vi "UHR-Fleezers Control (host) - 12.1.vi"() -> ()   [LabVIEW 2012] (continued)
            n683 = property on="Trap Pos. FB Offset Factor" class="DigNum (strict)"("Val(Sgnl)"=i64 0 ("Value (Signaling)")) -> ()  [unwired: 2 in, 2 out]
            n684 = local write "Stage Moving"(TRUE ("Stage Moving")) -> ()
            n685 = call "move to saved stage position.vi"("error in"=w1101, "Stage VISA resource name in"=w1102, "Position"="Stage Position To Establish FB", "Saved Stage Positions"=w1104) -> ("error out"=w1100:errorcluster)  [unwired: 1 out]
            n686 = local write "Stage Control Serial Error"(w1100) -> ()
          }
          frame #2 {
            n687 = call <vilib>:"Beep.vi"() -> ()  [unwired: 3 in, 9 out]
            n688 = Multiply(x="Wait (s)", y=u32 1000 ("milliseconds to wait")) -> (x*y=w1111:u32)
            n689 = property on="Trap Delta (MHz)" class="DigNum (strict)"("Val(Sgnl)"="Starting \nTrap Delta (MHz)") -> ()  [unwired: 2 in, 2 out]
            n690 = local write "Stage Moving"(FALSE ("Stage Moving")) -> ()
            n691 = Wait (ms)(milliseconds to wait=w1111) -> ()  [unwired: 1 out]
            n692 = property on="Tab Control 2" class="TabCtl (strict)"("Val(Sgnl)"=T6."Feedback on Trap Position" ("Value (Signaling)")) -> ()  [unwired: 2 in, 2 out]
            n693 = property on="Tab Control" class="TabCtl (strict)"("Val(Sgnl)"=T4."Trap Control (RF)" ("Value (Signaling)")) -> ()  [unwired: 2 in, 2 out]
          }
          frame #3 {
            n694 = property on="Set Reading to\nSetpoint" class="Bool (strict)"("Val(Sgnl)"=TRUE ("Value (Signaling)")) -> ()  [unwired: 2 in, 2 out]
            n695 = Wait (ms)(milliseconds to wait=u32 500) -> ()  [unwired: 1 out]
          }
          frame #4 {
            n696 = property on="Trap Pos. FB ON" class="Bool (strict)"("Val(Sgnl)"=TRUE ("Value (Signaling)")) -> ()  [unwired: 2 in, 2 out]
            n697 = Wait (ms)(milliseconds to wait=u32 250) -> ()  [unwired: 1 out]
          }
          frame #5 {
            n698 = case shown="False" "Trap Trig Fl." {
              frame False {
                n699 = case shown="True" "Green ON after FB ON?" {
                  selector: "Green ON after FB ON?" -> [_ w1126]
                  frame False {
                  }
                  frame True {
                    n700 = property on="Green Laser ON/Interlacing" class="Bool (strict)"("Val(Sgnl)"=w1126) -> ()  [unwired: 2 in, 2 out]
                  }
                }
              }
              frame True {
              }
            }
            n701 = case shown="True" "Remove Action Offset" {
              tunnel: TRUE ("Value (Signaling)") -> [w1123 w1124]
              frame False {
                n702 = property on="Remove Unwinding Offset" class="Bool (strict)"("Val(Sgnl)"=w1123) -> ()  [unwired: 2 in, 2 out]
              }
              frame True {
                n703 = property on="Remove Action Offset" class="Bool (strict)"("Val(Sgnl)"=w1124) -> ()  [unwired: 2 in, 2 out]
              }
            }
            n704 = Wait (ms)(milliseconds to wait=u32 250) -> ()  [unwired: 1 out]
          }
          frame #6 {
            n705 = property on="Start Saving" class="Bool (strict)"("Val(Sgnl)"=TRUE ("Value (Signaling)")) -> ()  [unwired: 2 in, 2 out]
            n706 = Wait (ms)(milliseconds to wait=u32 5000) -> ()  [unwired: 1 out]
          }
          frame #7 {
            w1130 = TRUE ("Value (Signaling)")
            n707 = property on="Rem fb disp offset" class="Bool (strict)"("Val(Sgnl)"=w1130) -> ()  [unwired: 2 in, 2 out]
            n708 = property on="Remove Offset" class="Bool (strict)"("Val(Sgnl)"=w1130) -> ()  [unwired: 2 in, 2 out]
            n709 = Wait (ms)(milliseconds to wait=u32 100) -> ()  [unwired: 1 out]
          }
          frame #8 {
            n710 = case shown="True" w1133 {
              frame False {
              }
              frame True {
                n711 = local write "Trap Trig. Fl."(TRUE ("Value (Signaling)")) -> ()
              }
            }
          }
          frame #9 {
            n712 = case shown="True" "Start dipping after?" {
              frame False {
              }
              frame True {
                n713 = flat-sequence {
                  frame #0 {
                    n714 = Multiply(x="Delay before dipping (s)", y=1000.0) -> (x*y=w1137:dbl)
                    n715 = Wait (ms)(milliseconds to wait=w1137) -> ()  [unwired: 1 out]
                  }
                  frame #1 {
                    n716 = property on="Dip for Protein" class="Bool (strict)"("Val(Sgnl)"=TRUE ("Value (Signaling)")) -> ()  [unwired: 2 in, 2 out]
                    n717 = local write "Scripts"(T1."Dipping" ("Scripts")) -> ()
                  }
                }
              }
            }
          }
        }
      }
      event "Fixed Traps Data\nScript": Value Change {
        n718 = event-data() -> ()  [unwired: 1 in, 5 out]
        n719 = flat-sequence {
          frame #0 {
            n720 = case shown="True" "Green ON" {
              frame False {
              }
              frame True {
                n721 = property on="Green Laser ON/Interlacing" class="Bool (strict)"("Val(Sgnl)"=TRUE) -> ()  [unwired: 2 in, 2 out]
              }
            }
            n722 = local write "Offset (nm)"(0.0 ("Offset (nm)")) -> ()
            n723 = property on="Sample Channel\nFlow" class="Bool (strict)"("Val(Sgnl)"=FALSE ("Value (Signaling)")) -> ()  [unwired: 2 in, 2 out]
            n724 = property on="Trap Delta (MHz)" class="DigNum (strict)"("Val(Sgnl)"="Fixed Traps Trap Delta (MHz)") -> ()  [unwired: 2 in, 2 out]
          }
          frame #1 {
            n725 = Wait (ms)(milliseconds to wait=u32 1000) -> ()  [unwired: 1 out]
          }
          frame #2 {
            n726 = local write "Start Saving"(TRUE ("Start Saving")) -> ()
          }
          frame #3 {
            n727 = local read "Bead Sep. Int. Time (s)"() -> (w1148:dbl)
            n728 = Multiply(x=w1148, y=1000.0) -> (x*y=w1150:dbl)
            n729 = Wait (ms)(milliseconds to wait=w1150) -> ()  [unwired: 1 out]
          }
          frame #4 {
            n730 = property on="Remove Offset" class="Bool (strict)"("Val(Sgnl)"=TRUE ("Value (Signaling)")) -> ()  [unwired: 2 in, 2 out]
          }
          frame #5 {
            n731 = property on="Dip for Protein" class="Bool (strict)"("Val(Sgnl)"="Start dipping after?") -> ()  [unwired: 2 in, 2 out]
          }
        }
      }
      event "Got DNA bead": Value Change {
        n732 = event-data() -> ()  [unwired: 1 in, 5 out]
        n733 = flat-sequence {
          frame #0 {
            n734 = local read "Daq spot flow on"() -> (w1155:bool)
            n735 = case shown="True" w1155 {
              frame False {
              }
              frame True {
                n736 = property on="Sample Channel\nFlow" class="Bool (strict)"("Val(Sgnl)"=TRUE ("Value (Signaling)")) -> ()  [unwired: 2 in, 2 out]
              }
            }
            n737 = property on="Got DNA bead" class="Bool"("Key Focus"=FALSE) -> ()  [unwired: 2 in, 2 out]
          }
          frame #1 {
            n738 = property on="Inject Pump 1" class="Bool (strict)"("Val(Sgnl)"=FALSE ("Value (Signaling)")) -> ()  [unwired: 2 in, 2 out]
          }
          frame #2 {
            n739 = property on="Cal/Data Acq. Spot" class="Bool (strict)"("Val(Sgnl)"=TRUE ("Value (Signaling)")) -> ()  [unwired: 2 in, 2 out]
          }
        }
      }
      event "Take Stepping Data": Value Change {
        n740 = event-data() -> ()  [unwired: 1 in, 5 out]
        n741 = local read "Save ave N"() -> (w1167:dbl)
        n742 = flat-sequence {
          tunnel: w1167 -> [w1169]
          tunnel: [w1169] -> w1162
          tunnel: [w1171] -> w1163
          tunnel: w1162 -> [w1171]
          tunnel: [w1173] -> w1164
          tunnel: w1163 -> [w1173]
          tunnel: [w1176] -> w1165
          tunnel: w1164 -> [w1176]
          tunnel: [w1178] -> w1166
          tunnel: w1165 -> [w1178]
          tunnel: [w1180] -> w1160
          tunnel: w1166 -> [w1180]
          tunnel: w1160 -> [w1183]
          tunnel: [w1183] -> w1159
          tunnel: w1159 -> [w1184]
          tunnel: [w1184] -> w1161
          tunnel: w1161 -> [w1190]
          frame #0 {
            n743 = property on="Save ave N" class="DigNum (strict)"("Val(Sgnl)"="Save ave factor") -> ()  [unwired: 2 in, 2 out]
          }
          frame #1 {
            n744 = Wait (ms)(milliseconds to wait=u32 100) -> ()  [unwired: 1 out]
          }
          frame #2 {
            n745 = local read "Offset 2 Start (MHz)"() -> (w1175:dbl)
            n746 = property on="Saved AOD Raster Scan Parameter Sets" class="Arr (strict)"("Index Values"=u32[] [2]) -> ()  [unwired: 2 in, 2 out]
            n747 = property on="Trap Delta (MHz)" class="DigNum (strict)"("Val(Sgnl)"=w1175) -> ()  [unwired: 2 in, 2 out]
          }
          frame #3 {
            n748 = property on="Load parameters" class="Bool (strict)"("Val(Sgnl)"=TRUE ("Value (Signaling)")) -> ()  [unwired: 2 in, 2 out]
          }
          frame #4 {
            n749 = Wait (ms)(milliseconds to wait=u32 100) -> ()  [unwired: 1 out]
          }
          frame #5 {
            n750 = property on="Trap Raster Scan" class="Bool (strict)"("Val(Sgnl)"=TRUE ("Value (Signaling)")) -> ()  [unwired: 2 in, 2 out]
          }
          frame #6 {
            n751 = Wait (ms)(milliseconds to wait=u32 1000) -> ()  [unwired: 1 out]
          }
          frame #7 {
            n752 = while {
              stop <- w1187 stop-if-true
              n753 = local read "Raster Scanning..."() -> (w1189:bool)
              n754 = local read "Saving..."() -> (w1188:bool)
              n755 = Not(x=w1188) -> (.not. x?=w1185:bool)
              n756 = Not(x=w1189) -> (.not. x?=w1186:bool)
              n757 = And(x=w1186, y=w1185) -> (x .and. y?=w1187:bool)
            }
          }
          frame #8 {
            n758 = property on="Save ave N" class="DigNum (strict)"("Val(Sgnl)"=w1190) -> ()  [unwired: 2 in, 2 out]
          }
        }
      }
      event "Step Size (nm)": Value Change {
        n759 = event-data() -> ()  [unwired: 1 in, 5 out]
        n760 = flat-sequence {
          frame #0 {
            n761 = property on="Saved AOD Raster Scan Parameter Sets" class="Arr (strict)"("Index Values"=u32[] [1]) -> ()  [unwired: 2 in, 2 out]
          }
          frame #1 {
            n762 = Multiply(x="N Steps", y="Step Size (nm)") -> (x*y=w1192:dbl)
            n763 = property on="Scan Speed AOD (nm/s) 2" class="DigNum (strict)"("Value"="Step Size (nm)") -> ()  [unwired: 2 in, 2 out]
            n764 = property on="Step Size AOD (nm) 2" class="DigNum (strict)"("Value"="Step Size (nm)") -> ()  [unwired: 2 in, 2 out]
            n765 = property on="Scan Range AOD (nm) 2" class="DigNum (strict)"("Value"=w1192) -> ()  [unwired: 2 in, 2 out]
          }
        }
      }
      event "Take Detection Laser\nImage": Value Change {
        n766 = event-data() -> ()  [unwired: 1 in, 5 out]
        n767 = flat-sequence {
          tunnel: [w1220] -> w1210
          tunnel: [w1219] -> w1203
          tunnel: [w1218] -> w1195
          tunnel: [w1223] -> w1211
          tunnel: w1210 -> [w1223]
          tunnel: [w1222] -> w1204
          tunnel: w1203 -> [w1222]
          tunnel: [w1221] -> w1196
          tunnel: w1195 -> [w1221]
          tunnel: [w1227] -> w1212
          tunnel: w1211 -> [w1227]
          tunnel: [w1226] -> w1205
          tunnel: w1204 -> [w1226]
          tunnel: [w1225] -> w1197
          tunnel: w1196 -> [w1225]
          tunnel: [w1233] -> w1213
          tunnel: w1212 -> [w1233]
          tunnel: [w1232] -> w1206
          tunnel: w1205 -> [w1232]
          tunnel: [w1231] -> w1198
          tunnel: w1197 -> [w1231]
          tunnel: [w1237] -> w1214
          tunnel: w1213 -> [w1237]
          tunnel: [w1236] -> w1207
          tunnel: w1206 -> [w1236]
          tunnel: [w1235] -> w1199
          tunnel: w1198 -> [w1235]
          tunnel: [w1241] -> w1215
          tunnel: w1214 -> [w1241]
          tunnel: [w1240] -> w1208
          tunnel: w1207 -> [w1240]
          tunnel: [w1239] -> w1200
          tunnel: w1199 -> [w1239]
          tunnel: [w1245] -> w1216
          tunnel: w1215 -> [w1245]
          tunnel: [w1244] -> w1209
          tunnel: w1208 -> [w1244]
          tunnel: [w1243] -> w1201
          tunnel: w1200 -> [w1243]
          tunnel: w1216 -> [w1251]
          tunnel: w1209 -> [w1250]
          tunnel: [w1248] -> w1202
          tunnel: w1201 -> [w1248]
          tunnel: w1202 -> [w1252]
          frame #0 {
            n768 = local read "Green Laser ON/Interlacing"() -> (w1220:bool)
            n769 = local read "Green laser mode"() -> (w1219:enum32{"Laser ON", "Laser OFF", "Interlace"})
            n770 = local read "Green FB On/Off"() -> (w1218:bool)
          }
          frame #1 {
            n771 = property on="Green FB On/Off" class="Bool (strict)"("Val(Sgnl)"=FALSE ("Value (Signaling)")) -> ()  [unwired: 2 in, 2 out]
          }
          frame #2 {
            n772 = property on="Green Laser ON/Interlacing" class="Bool (strict)"("Val(Sgnl)"=TRUE ("Value (Signaling)")) -> ()  [unwired: 2 in, 2 out]
            n773 = property on="Flip Green Filter" class="Bool (strict)"("Val(Sgnl)"=TRUE ("Value (Signaling)")) -> ()  [unwired: 2 in, 2 out]
            n774 = property on="Green laser mode" class="RadioBtnsControl (strict)"("Val(Sgnl)"=enum32{"Laser ON", "Laser OFF", "Interlace"}."Laser ON" ("Value (Signaling)")) -> ()  [unwired: 2 in, 2 out]
          }
          frame #3 {
            n775 = Wait (ms)(milliseconds to wait=u32 500) -> ()  [unwired: 1 out]
          }
          frame #4 {
            n776 = property on="Confocal Image" class="Bool (strict)"("Val(Sgnl)"=TRUE ("Value (Signaling)")) -> ()  [unwired: 2 in, 2 out]
          }
          frame #5 {
            n777 = Wait (ms)(milliseconds to wait=u32 2000) -> ()  [unwired: 1 out]
          }
          frame #6 {
            n778 = while {
              stop <- w1246 stop-if-true
              n779 = local read "Saving..."() -> (w1247:bool)
              n780 = Not(x=w1247) -> (.not. x?=w1246:bool)
            }
          }
          frame #7 {
            n781 = property on="Flip Green Filter" class="Bool (strict)"("Val(Sgnl)"=TRUE ("Value (Signaling)")) -> ()  [unwired: 2 in, 2 out]
            n782 = property on="Green Laser ON/Interlacing" class="Bool (strict)"("Val(Sgnl)"=w1251) -> ()  [unwired: 2 in, 2 out]
            n783 = property on="Green laser mode" class="RadioBtnsControl (strict)"("Val(Sgnl)"=w1250) -> ()  [unwired: 2 in, 2 out]
          }
          frame #8 {
            n784 = property on="Green FB On/Off" class="Bool (strict)"("Val(Sgnl)"=w1252) -> ()  [unwired: 2 in, 2 out]
          }
        }
      }
      event "Stop All": Value Change {
        n785 = event-data() -> ()  [unwired: 1 in, 5 out]
        n786 = local read "Stop All"() -> (w1253:bool)
      }
    }
    n787 = node-c288() -> ()  [unwired: 1 in, 1 out]
  }
  n788 = node-c288(3 ("Processor")) -> (w114:T20)  [unwired: 3 out]
  n789 = flat-sequence "Video" {
    tunnel: [w1263] -> w104
    tunnel: w104 -> [w1303]
    frame #0 {
      n790 = while {
        stop <- w1255 continue-if-true
        n791 = call "Close Video Capture.vi"() -> ("error code OUT"=w1257:i32)
        n792 = Equal?(x=w1257, y=0) -> (x = y?=w1255:bool)
      }
      n793 = local write "Stop All"(FALSE ("Stop All")) -> ()
    }
    frame #1 {
      n794 = call "DMR_Init.vi"() -> ()  [unwired: 3 out]
    }
    frame #2 {
      w1258 = "DE245428202"  # MSU fleezers card #
      (unwired) "DE019116701"  # Illinois fleezers card #
      # "Setting the destination format to Mono8 makes sure that the image can be displayed in the intensity plot."
      n795 = call "DMR_GetDevice.vi"("search string IN"=w1258) -> ("device handle OUT"=w1281:i32)  [unwired: 4 in, 2 out]
      n796 = call "DMR_OpenDevice.vi"("device handle IN"=w1281) -> ("driver handle OUT"=w1264:i32)  [unwired: 4 out]
      n797 = call "DMR_FindList.vi"("flags IN"=u32 0 ("flags"), "list name IN"="" ("String"), "list type IN"=T25."camera descriptions", "driver handle IN"=w1264) -> ("list handle OUT"=w1267:i32)  [unwired: 2 out]
      n798 = call "DMR_FindList.vi"("flags IN"=u32 0 ("flags"), "list name IN"="Base", "list type IN"=T25."setting", "driver handle IN"=w1264) -> ("list handle OUT"=w1265:i32)  [unwired: 2 out]
      n799 = call "OBJ_GetHandle.vi"("object name IN"="VideoStandard", "list handle IN"=w1267) -> ("object handle OUT"=w1261:i32)  [unwired: 3 out]
      n800 = call "OBJ_GetHandle.vi"("object name IN"="PixelFormat", "list handle IN"=w1265) -> ("object handle OUT"=w1275:i32)  [unwired: 3 out]
      n801 = call "OBJ_SetS.vi"("value index IN"=0, "value IN"="NTSC M", "object handle IN"=w1261) -> ()  [unwired: 2 out]
      n802 = call "OBJ_SetS.vi"("value index IN"=0, "value IN"="Mono8" ("value"), "object handle IN"=w1275) -> ()  [unwired: 2 out]
      n803 = call "OBJ_GetHandle.vi"("object name IN"="VideoChannel", "list handle IN"=w1265) -> ("object handle OUT"=w1271:i32)  [unwired: 3 out]
      n804 = while {
        tunnel: [w1285] -> w1263
        tunnel: w1264 -> [w1282]
        stop <- w1283 continue-if-true
        n805 = call "DMR_ImageRequestSingle.vi"("request control IN"=0, "driver handle IN"=w1282) -> ("error code OUT"=w1284:i32, "driver handle OUT"=w1285:i32)  [unwired: 2 out]
        n806 = Equal To 0?(x=w1284) -> (x = 0?=w1283:bool)
      }
      n807 = call "OBJ_SetI.vi"("value index IN"=0, "value IN"=3 ("Video channel"), "object handle IN"=w1271) -> ()  [unwired: 2 out]
    }
    frame #3 {
      w1291 = T16 0 items=["Grayscale (U8)", "Grayscale (I16)", "Grayscale (SGL)", "Complex (CSG)", "RGB (U32)", "HSL (U32)", "RGB (U64)"] ("Image Type")
      w1299 = T16 0 items=["Grayscale (U8)", "Grayscale (I16)", "Grayscale (SGL)", "Complex (CSG)", "RGB (U32)", "HSL (U32)", "RGB (U64)"] ("Image Type")
      n808 = for "Create Greyscale map" {
        N: 256 -> [_]
        tunnel: [w1305] -> w1288 mode=indexing
        workers-P: _ -> [_]
        i -> [w1308]
        n809 = To Unsigned Byte Integer(number=w1308) -> (unsigned 8bit integer=w1304:u8)
        n810 = Join Numbers(hi=w1304, lo=w1304) -> ((hi.lo)=w1307:u16)
        n811 = Join Numbers(hi=w1304, lo=w1304) -> ((hi.lo)=w1306:u16)
        n812 = Join Numbers(hi=w1307, lo=w1306) -> ((hi.lo)=w1305:u32)
      }
      n813 = call "IMAQ Create"("Image Name"="Scaled video", "Image Type"=w1291) -> ("New Image"=w1290:T2)  [unwired: 2 in, 2 out]
      n814 = call "IMAQ Create"("Image Name"="Main video", "Image Type"=w1299) -> ("New Image"=w1300:T2)  [unwired: 2 in, 2 out]
      n815 = node-c288(0 ("Processor")) -> (w1298:T20)  [unwired: 3 out]
      n816 = Initialize Array(u32 0 ("Window Number (0...15)"), 480 ("dimension size"), 640 ("dimension size")) -> (w1293:u32[][])
      n817 = timed-loop {
        tunnel: w1303 -> [w1325]
        tunnel: [w1324] -> w1302
        tunnel: w1300 -> [w1323]
        timing: w1298 -> [_]
        timing-out: [_] -> w1297
        tunnel: w1293 -> [w1312]
        tunnel: w1290 -> [w1310]
        tunnel: w1288 -> [w1309]
        stop <- w1311 stop-if-true
        # "This block performs the \nactual image capture."
        n818 = node-c288() -> ()  [unwired: 2 out]
        n819 = local read "Stop All"() -> (w1311:bool)
        n820 = Reciprocal(x="Video Capture Rate (Hz)") -> (1/x=w1315:dbl)
        n821 = Multiply(x=w1315, y=1000.0) -> (x*y=w1313:dbl)
        n822 = call "DMR_ImageRequestWaitFor.vi"("queue number IN"=0, "timeout(ms) IN"=500, "driver handle IN"=w1325) -> ("error code OUT"=w1329:i32, "request number OUT"=w1326:i32, "driver handle OUT"=w1327:i32)
        n823 = feedback #1(T26 refnum ("Avi Refnum")) -> (w1317:T26)
        n824 = case shown="True" "New Video File" {
          tunnel: [T26 refnum ("Avi Refnum") w1346] -> w1319
          tunnel: [FALSE TRUE] -> w1320
          tunnel: w1317 -> [_ w1342]
          frame False {
          }
          frame True {
            n825 = call "Create new save file.vi"("Ext"=".avi" ("string"), "Index In"="Video Index") -> ("Path Out"=w1338:path, "Index Out"=w1339:dbl)  [unwired: 1 in]
            "Path Out" <- w1338
            n826 = Not Equal?(x=w1342, y=T26 refnum ("Avi Refnum")) -> (x != y?=w1343:bool)
            n827 = Increment(x=w1339) -> (x+1=w1348:dbl)
            n828 = case shown="True" w1343 {
              tunnel: w1342 -> [_ w1349]
              frame False {
              }
              frame True {
                n829 = call "IMAQ AVI Close"("Avi Refnum"=w1349) -> ()  [unwired: 1 in, 10 out]
              }
            }
            n830 = local write "Video Index"(w1348) -> ()
            n831 = call "IMAQ AVI Create"("Frames Per Second"=u32 30, "AVI Path"=w1338) -> ("Avi Refnum"=w1346:T26)  [unwired: 5 in, 4 out]
          }
        }
        n832 = Equal To 0?(x=w1329) -> (x = 0?=w1328:bool)
        n833 = Select(t=w1319, s=w1320, f=w1317) -> (s? t:f=w1318:T26)
        n834 = feedback-in #1(w1318) -> ()
        n835 = case shown="True" w1328 {
          tunnel: w1327 -> [w1350 w1375]
          tunnel: w1326 -> [_ w1374]
          tunnel: [w1350 w1371] -> w1324
          tunnel: w1323 -> [_ w1355]
          tunnel: w1312 -> [_ w1359]
          tunnel: w1318 -> [_ w1357]
          tunnel: w1310 -> [_ w1352]
          tunnel: w1309 -> [_ w1351]
          frame False {
          }
          frame True {
            w1365 = u32 0 ("X-offset IN")
            n836 = call "DMR_GetImageRequestBufferData.vi"("driver handle IN"=w1375, "request number IN"=w1374) -> ("width OUT"=w1364:i32, "height OUT"=w1363:i32, "driver handle OUT"=w1370:i32, "request number OUT"=w1369:i32, "bytes per pixel OUT"=w1366:i32)  [unwired: 13 out]
            n837 = call "DMR_GetImageRequestBufferImageData.vi"("driver handle IN"=w1370, "request number IN"=w1369, "bytes per pixel IN"=w1366, "X-offset IN"=w1365, "Y-offset IN"=w1365, "height IN"=w1363, "width IN"=w1364) -> ("driver handle OUT"=w1368:u32, "request number OUT"=w1367:u32, "image OUT"=w1360:u32[][])  [unwired: 10 out]
            n838 = call "DMR_ImageRequestUnlock.vi"("request number IN"=w1367, "driver handle IN"=w1368) -> ("driver handle OUT"=w1373:i32)  [unwired: 1 in, 2 out]
            n839 = case shown="True" "Averaging" {
              tunnel: w1360 -> [w1411 w1416]
              tunnel: [w1411 w1415] -> w1356
              tunnel: w1359 -> [_ w1413]
              frame False {
              }
              frame True {
                (unwired) 1
                w1421 = 1
                n840 = feedback #2(w1413) -> (w1412:u32[][])
                n841 = Add(x=w1416, y=w1412) -> (x+y=w1417:u32[][])
                n842 = Select(t=w1413, s="Reset Averaging", f=w1417) -> (s? t:f=w1419:u32[][])
                n843 = feedback-in #2(w1419) -> ()
                n844 = feedback #3(w1421) -> (w1414:i32)
                n845 = Divide(x=w1417, y=w1414) -> (x/y=w1418:dbl[][])
                n846 = Increment(x=w1414) -> (x+1=w1422:i32)
                n847 = To Unsigned Long Integer(number=w1418) -> (unsigned 32bit integer=w1415:u32[][])
                n848 = Select(t=w1421, s="Reset Averaging", f=w1422) -> (s? t:f=w1420:i32)
                n849 = feedback-in #3(w1420) -> ()
              }
            }
            n850 = call "DMR_ImageRequestSingle.vi"("request control IN"=0, "driver handle IN"=w1373) -> ("driver handle OUT"=w1371:i32)  [unwired: 3 out]
            n851 = disable-structure shown="Disabled" {
              disable-tunnel: w1356 -> [w1388 _]
              disable-tunnel: w1352 -> [w1387 _]
              frame Disabled {
                n852 = To Double Precision Float(number=w1388) -> (double precision float=w1386:dbl[][])
                n853 = In Range and Coerce(upper limit="Intensity Upper", x=w1386, lower limit="Intensity Lower") -> (coerced(x)=w1385:dbl[][])  [unwired: 1 out]
                n854 = Subtract(x="Intensity Upper", y="Intensity Lower") -> (x-y=w1382:dbl)
                n855 = Subtract(x=w1385, y="Intensity Lower") -> (x-y=w1383:dbl[][])
                n856 = Divide(x=w1383, y=w1382) -> (x/y=w1384:dbl[][])
                n857 = Multiply(x=255.0, y=w1384) -> (x*y=w1380:dbl[][])
                n858 = To Unsigned Byte Integer(number=w1380) -> (unsigned 8bit integer=w1389:u8[][])
                n859 = call "IMAQ ArrayToImage"("Image Pixels (U8)"=w1389, "Image"=w1387) -> ("Image Out"=w1376:T2)  [unwired: 4 in, 5 out]
                n860 = First Call?() -> (First Call?: T/F=w1377:bool)
                n861 = case shown="True" w1377 {
                  tunnel: w1376 -> [w1390 w1401]
                  frame False {
                    n862 = flat-sequence {
                      tunnel: w1390 -> [w1396]
                      frame #0 {
                        w1393 = FALSE ("Get/Set Status? (Set)")
                        w1392 = 0 ("Window Number (0...15)")
                        n863 = call "IMAQ WindSize"("Get/Set Status? (Set)"=w1393, "Window Number"=w1392) -> ("Width & Height out"=→"Window Size":cluster{"Width":i32, "Height":i32})  [unwired: 4 in, 2 out]
                        n864 = call "IMAQ WindMove"("Window Number (0...15)"=w1392, "Get/Set Status? (Set)"=w1393) -> ("Coordinates (screen)"=→"Window Position":cluster{"X Position":i32, "Y Position":i32})  [unwired: 3 in, 1 out]
                        n865 = call "IMAQ WindDraw"("Resize to Image Size? (Y)"=FALSE, "Window Number (0...15)"=w1392, "Image"=w1396) -> ()  [unwired: 7 in, 2 out]
                      }
                      frame #1 {
                        n866 = call "IMAQ WindZoom 2"("Center Point"="Center Point", "Zoom to Fit? (False)"=FALSE, "Zoom Factor"="Zoom Factor") -> ()  [unwired: 5 in, 4 out]
                      }
                    }
                  }
                  frame True {
                    n867 = flat-sequence {
                      tunnel: w1401 -> [w1404]
                      tunnel: [w1402] -> w1400
                      tunnel: w1400 -> [w1406]
                      frame #0 {
                        w1403 = TRUE ("Resize to Image Size? (Y)")
                        w1402 = 0 ("Window Number (0...15)")
                        n868 = call "IMAQ WindNonTearing"("Window Number"=w1402, "NonTearing? (True)"=w1403) -> ()  [unwired: 8 in, 2 out]
                        n869 = call "IMAQ WindDraw"("Resize to Image Size? (Y)"=w1403, "Window Number (0...15)"=w1402, "Image"=w1404) -> ()  [unwired: 7 in, 2 out]
                      }
                      frame #1 {
                        n870 = call "IMAQ WindSize"("Scrollbars? (N)"=FALSE, "Width & Height"="Initial Window Size", "Window Number"=w1406) -> ()  [unwired: 3 in, 3 out]
                        n871 = call "IMAQ WindMove"("Window Number (0...15)"=w1406, "Coordinates (screen)"="Initial Window Position") -> ()  [unwired: 3 in, 2 out]
                      }
                    }
                  }
                }
              }
              frame Enabled {
              }
            }
            n872 = To Unsigned Byte Integer(number=w1356) -> (unsigned 8bit integer=w1354:u8[][])
            n873 = call "IMAQ ArrayToImage"("Image Pixels (U8)"=w1354, "Image"=w1355) -> ("Image Out"=w1353:T2)  [unwired: 4 in, 5 out]
            "Primary Video Display" <- w1353
            n874 = case shown="True" "Save Video" {
              tunnel: w1357 -> [_ w1410]
              tunnel: w1353 -> [_ w1409]
              frame False {
              }
              frame True {
                n875 = call "IMAQ AVI Write Frame"("Image"=w1409, "Avi Refnum"=w1410) -> ()  [unwired: 2 in, 8 out]
              }
            }
            n876 = case shown="True" "Save Image" {
              tunnel: w1354 -> [_ w1425]
              tunnel: w1351 -> [_ w1424]
              frame False {
              }
              frame True {
                n877 = call <vilib>:"Flatten Pixmap.vi"("colors"=w1424, "8-bit pixmap"=w1425) -> ("image data"=w1431:T27)  [unwired: 4 in, 5 out]
                n878 = call "Create new save file.vi"("Insert"="video_frame_" ("string"), "Ext"=".bmp" ("string"), "Index In"="Image Index") -> ("Path Out"=w1427:path, "Index Out"=w1432:dbl)
                n879 = Increment(x=w1432) -> (x+1=w1426:dbl)
                n880 = local write "Image Index"(w1426) -> ()
                n881 = call <vilib>:"Write BMP File.vi"("image data"=w1431, "path to BMP file"=w1427) -> ()  [unwired: 1 in, 9 out]
              }
            }
          }
        }
        n882 = node-c288(w1313) -> ()  [unwired: 1 out]
      }
      n883 = node-c288(w1297) -> ()  [unwired: 1 out]
      n884 = call "DMR_CloseDevice.vi"("driver handle IN"=w1302) -> ()  [unwired: 1 in, 4 out]
    }
    frame #4 {
      n885 = call "DMR_Close.vi"() -> ()  [unwired: 1 out]
    }
  }
  n886 = timed-loop "Acquire Data" {
    tunnel: w28 -> [w1724]
    tunnel: w76 -> [w1723]
    tunnel: [w1753] -> w286
    tunnel: [w1748] -> w284
    timing: w194 -> [_]
    timing-out: [_] -> w193
    tunnel: w93 -> [w1569]
    stop <- "Stop All" stop-if-true
    w1484 = "Initialize"
    w1554 = "NI_ChannelName" ("name")
    n887 = node-c288() -> ()  [unwired: 2 out]
    n888 = First Call?() -> (First Call?: T/F=w1519:bool)
    n889 = Or(x="Reset", y=w1519) -> (x .or. y?=w1520:bool)
    n890 = local read "Flushing P1"() -> (w1439:bool)
    n891 = case "Reset data stream" shown="True" w1520 {
      tunnel: w1724 -> [w2729 w2737]
      tunnel: w1723 -> [w2728 w2736]
      tunnel: [w2729 w2731] -> w1719
      tunnel: [w2728 w2730] -> w1718
      frame False {
      }
      frame True {
        w2734 = TRUE ("AI to FIFO")
        n892 = local write "Overflow (data lost)"(FALSE ("Overflow (data lost)")) -> ()
        n893 = call "reset FPGA DMA.vi"("error in"=w2736, "FPGA VI Reference In"=w2737) -> ("error out"=w2732:errorcluster, "FPGA VI Reference Out"=w2733:T18)
        n894 = xnode "Read/Write Control"("FPGA VI Reference In"=w2733, "error in"=w2732, "AI to FIFO"=w2734, "APD to FIFO"=w2734) -> ("FPGA VI Reference Out"=w2731:T18, "error out"=w2730:errorcluster)
      }
    }
    n895 = case shown="True" w1439 {
      frame False {
      }
      frame True {
        n896 = local read "Flush rate (uL/m) P1"() -> (w1770:dbl)
        n897 = local read "HP1 Flush Time (s)"() -> (w1779:dbl)
        n898 = local read "DMA Update Period (s)"() -> (w1773:dbl)
        n899 = Divide(x=w1770, y=60.0) -> (x/y=w1771:dbl)
        n900 = Divide(x=w1779, y=w1773) -> (x/y=w1768:dbl)
        n901 = feedback #4(0) -> (w1777:i32)
        n902 = Increment(x=w1777) -> (x+1=w1767:i32)
        n903 = Greater?(x=w1767, y=w1768) -> (0:w1776:bool)
        n904 = Compound Arithmetic op=MULTIPLY(w1773, w1767, w1771) -> (→"P1 Flush Volume (uL)":dbl)
        n905 = Divide(x=w1767, y=w1768) -> (x/y=→"P1 Flushing Bar":dbl)
        n906 = case shown="True" w1776 {
          tunnel: w1767 -> [w1780 _]
          tunnel: [w1780 0] -> w1775
          frame False {
          }
          frame True {
            w1781 = FALSE ("Flushing P1")
            n907 = local write "Inject Pump 1"(w1781) -> ()
            n908 = local write "Flushing P1"(w1781) -> ()
            n909 = property on="Clear Volume P1" class="Bool (strict)"("Val(Sgnl)"=TRUE ("Value (Signaling)")) -> ()  [unwired: 2 in, 2 out]
          }
        }
        n910 = feedback-in #4(w1775) -> ()
      }
    }
    n911 = Or(x="Start AOD Scan", y="Trap Raster Scan") -> (x .or. y?=w1675:bool)
    n912 = case "Start AOM raster scan" shown="True" w1675 {
      tunnel: w1719 -> [w2579 w2589]
      tunnel: w1718 -> [w2578 w2588]
      tunnel: [w2579 w2582] -> w1717
      tunnel: [w2578 w2581] -> w1716
      frame False {
      }
      frame True {
        n913 = case shown="True" "Restart DMA? (AOD)" {
          tunnel: [w2627 w2629] -> w2583
          tunnel: [w2626 w2628] -> w2584
          tunnel: w2589 -> [w2627 w2631]
          tunnel: w2588 -> [w2626 w2630]
          frame False {
          }
          frame True {
            n914 = local write "Overflow (data lost)"(FALSE ("Overflow (data lost)")) -> ()
            n915 = call "reset FPGA DMA.vi"("error in"=w2630, "FPGA VI Reference In"=w2631) -> ("error out"=w2628:errorcluster, "FPGA VI Reference Out"=w2629:T18)
          }
        }
        n916 = local write "Trap Raster Scan"(FALSE ("Trap Raster Scan")) -> ()
        n917 = case shown="True" "Move MCL Also?" {
          tunnel: w2584 -> [w2592 w2621]
          tunnel: w2583 -> [w2593 w2622]
          tunnel: [w2591 w2625] -> w2582
          tunnel: [w2590 w2624] -> w2581
          frame False {
            w2594 = TRUE ("AI to FIFO")
            n918 = xnode "Read/Write Control"("FPGA VI Reference In"=w2593, "error in"=w2592, "AI to FIFO"=w2594, "APD to FIFO"=w2594, "Start scan"=w2594) -> ("FPGA VI Reference Out"=w2591:T18, "error out"=w2590:errorcluster)
          }
          frame True {
            w2618 = FALSE ("1D or 2D Scan?")
            w2623 = TRUE ("AI to FIFO")
            # "Count for MCL loop"
            # "N total cycles"
            # "N steps"
            # "V_int"
            n919 = local read "Scan Range (nm)"() -> (w2600:dbl)
            n920 = local read "Number of F/B Scans (AOD)"() -> (w2617:u16)
            n921 = Sign(1:w2600) -> (0:w2599:dbl)
            n922 = Compound Arithmetic op=MULTIPLY(w2600, "MCL Step Position Ratio", "MCL/AOM Scale Tweak") -> (w2604:dbl)
            n923 = Negate(x=w2599) -> (-x=w2596:dbl)
            n924 = Multiply(x=w2596, y="MCL Step Increment (V_int)") -> (x*y=w2598:dbl)
            n925 = Divide(x=w2604, y="MCL X Cal (nm/V)") -> (x/y=w2610:dbl)
            n926 = Multiply(x=32767.0 ("y"), y=w2610) -> (x*y=w2616:dbl)
            n927 = local read "Total Counts (ticks)"() -> (w2601:u32)
            n928 = local read "Cycles/step (AOD)"() -> (w2612:u64)
            n929 = local read "Scan steps (AOD)"() -> (w2613:u64)
            n930 = Divide(x=w2616, y=10.0) -> (x/y=w2609:dbl)
            n931 = Divide(x=w2609, y="MCL Step Increment (V_int)") -> (x/y=w2607:dbl)
            n932 = Absolute Value(x=w2607) -> (abs(x)=w2595:dbl)
            n933 = Compound Arithmetic op=MULTIPLY(w2613, w2612, w2601) -> (w2608:u64)
            n934 = local write "wait to reset values"(w2623) -> ()
            n935 = local write "MCL Scanning"(w2623) -> ()
            n936 = Divide(x=w2608, y=w2595) -> (x/y=w2605:dbl)
            "MCL Count" <- w2605
            n937 = xnode "Read/Write Control"("FPGA VI Reference In"=w2622, "error in"=w2621, "Scan steps (MCL)"=w2595, "Number of scans (MCL)"=w2617, "Cycles per step (MCL)"=u64 1, "Scan freq.  increment (MCL)"=w2598, "1D or 2D Scan?"=w2618, "MCL Scan Axis"=w2618, "Cont. Scan (MCL)"=w2618, "MCL count"=w2605) -> ("FPGA VI Reference Out"=w2620:T18, "error out"=w2619:errorcluster)
            n938 = xnode "Read/Write Control"("FPGA VI Reference In"=w2620, "error in"=w2619, "AI to FIFO"=w2623, "APD to FIFO"=w2623, "Start scan"=w2623, "Start scan (MCL)"=w2623) -> ("FPGA VI Reference Out"=w2625:T18, "error out"=w2624:errorcluster)
          }
        }
        "Raster Scanning..." <- TRUE ("Scanning...")
      }
    }
    n939 = local read "Flushing P3"() -> (w1440:bool)
    n940 = case "Keep track of when Harvard Pump 3 is done flushing" shown="True" w1440 {
      frame False {
      }
      frame True {
        n941 = local read "Flush rate (uL/m) P3"() -> (w1787:dbl)
        n942 = local read "DMA Update Period (s)"() -> (w1789:dbl)
        n943 = local read "HP3 Flush Time (s)"() -> (w1796:dbl)
        n944 = Divide(x=w1787, y=60.0) -> (x/y=w1785:dbl)
        n945 = feedback #5(0) -> (w1794:i32)
        n946 = Increment(x=w1794) -> (x+1=w1788:i32)
        n947 = Divide(x=w1796, y=w1789) -> (x/y=w1790:dbl)
        n948 = Greater?(x=w1788, y=w1790) -> (0:w1793:bool)
        n949 = Compound Arithmetic op=MULTIPLY(w1789, w1788, w1785) -> (→"P3 Flush Volume (uL)":dbl)
        n950 = case shown="True" w1793 {
          tunnel: w1788 -> [w1797 _]
          tunnel: [w1797 0] -> w1792
          frame False {
          }
          frame True {
            w1798 = FALSE ("Flushing P3")
            n951 = local write "Inject Pump 3"(w1798) -> ()
            n952 = local write "Flushing P3"(w1798) -> ()
            n953 = property on="Clear Volume P3" class="Bool (strict)"("Val(Sgnl)"=TRUE ("Value (Signaling)")) -> ()  [unwired: 2 in, 2 out]
          }
        }
        n954 = feedback-in #5(w1792) -> ()
        n955 = Divide(x=w1788, y=w1790) -> (x/y=→"P3 Flushing Bar":dbl)
      }
    }
    n956 = And(x="Save scans", y=w1675) -> (x .and. y?=w1715:bool)
    n957 = Compound Arithmetic op=OR("Start MCL Scan", "Confocal Image", "Confocal Linescan") -> (w1673:bool)
    n958 = And(x="Save Data (MCL)", y=w1673) -> (x .and. y?=w1714:bool)
    n959 = case "Start MCL raster scan" shown="True" w1673 {
      tunnel: w1717 -> [w2196 w2212]
      tunnel: w1716 -> [w2195 w2211]
      tunnel: [w2196 w2207] -> w1567
      tunnel: [w2195 w2206] -> w1566
      tunnel: [FALSE w2205] -> w1700
      tunnel: "Start MCL Scan" -> [_ w2200]
      tunnel: "Confocal Image" -> [_ w2199]
      tunnel: "Confocal Linescan" -> [_ _]
      frame False {
      }
      frame True {
        w2205 = TRUE
        n960 = case shown="True" "Restart DMA? (MCL)" {
          tunnel: [w2257 w2259] -> w2210
          tunnel: [w2256 w2258] -> w2209
          tunnel: w2212 -> [w2257 w2262]
          tunnel: w2211 -> [w2256 w2261]
          frame False {
          }
          frame True {
            n961 = call "reset FPGA DMA.vi"("error in"=w2261, "FPGA VI Reference In"=w2262) -> ("error out"=w2258:errorcluster, "FPGA VI Reference Out"=w2259:T18)
            n962 = local write "Overflow (data lost)"(FALSE ("Overflow (data lost)")) -> ()
          }
        }
        n963 = case shown="False" w2200 {
          selector: w2200 -> [_ w2216]
          tunnel: w2199 -> [w2215 _]
          tunnel: [w2215 w2216] -> w2198
          frame False {
            n964 = property on="2D or 1D Scan" class="Bool (strict)"("Val(Sgnl)"=w2215) -> ()  [unwired: 2 in, 2 out]
            n965 = property on="Confocal Image" class="Bool (strict)"("Value"=FALSE ("Start Confocal Map")) -> ()  [unwired: 2 in, 2 out]
          }
          frame True {
          }
        }
        n966 = local write "MCL Scanning"(w2205) -> ()
        n967 = local read "AO1"() -> (w2202:dbl)
        n968 = local read "AO2"() -> (w2201:dbl)
        n969 = case shown="True" "Center Scan" {
          tunnel: w2210 -> [w2223 w2255]
          tunnel: w2209 -> [w2222 w2254]
          tunnel: [w2221 w2253] -> w2207
          tunnel: [w2220 w2252] -> w2206
          tunnel: [w2218 w2239] -> w2204
          tunnel: [w2217 w2238] -> w2203
          tunnel: w2202 -> [w2218 w2244]
          tunnel: w2201 -> [w2217 w2247]
          tunnel: w2198 -> [_ _]
          frame False {
            w2219 = TRUE ("AI to FIFO")
            n970 = xnode "Read/Write Control"("FPGA VI Reference In"=w2223, "error in"=w2222, "AI to FIFO"=w2219, "APD to FIFO"=w2219, "Start scan (MCL)"=w2219) -> ("FPGA VI Reference Out"=w2221:T18, "error out"=w2220:errorcluster)
          }
          frame True {
            w2251 = TRUE ("AI to FIFO")
            n971 = local read "Scan steps (MCL)"() -> (w2230:u64)
            n972 = local read "Scan lines (y)"() -> (w2226:u64)
            n973 = local read "Fast Scan Dir"() -> (w2237:bool)
            n974 = local read "Actual MCL Inc (V)"() -> (w2227:dbl)
            n975 = Decrement(x=w2226) -> (x-1=w2225:u64)
            n976 = Decrement(x=w2230) -> (x-1=w2229:u64)
            n977 = Multiply(x=w2227, y=w2225) -> (x*y=w2224:dbl)
            n978 = Divide(x=w2224, y=2.0) -> (x/y=w2234:dbl)
            n979 = Multiply(x=w2227, y=w2229) -> (x*y=w2228:dbl)
            n980 = Divide(x=w2228, y=2.0) -> (x/y=w2233:dbl)
            n981 = Select(t=w2233, s=w2237, f=w2234) -> (s? t:f=w2232:dbl)
            n982 = Select(t=w2234, s=w2237, f=w2233) -> (s? t:f=w2236:dbl)
            n983 = Subtract(x=w2244, y=w2236) -> (x-y=w2235:dbl)
            n984 = Subtract(x=w2247, y=w2232) -> (x-y=w2231:dbl)
            n985 = local read "2D or 1D Scan"() -> (w2249:bool)
            n986 = Not(x=w2237) -> (.not. x?=w2243:bool)
            n987 = Not(x=w2249) -> (.not. x?=w2245:bool)
            n988 = And(x=w2237, y=w2245) -> (x .and. y?=w2246:bool)
            n989 = And(x=w2245, y=w2243) -> (x .and. y?=w2248:bool)
            n990 = Select(t=w2247, s=w2248, f=w2231) -> (s? t:f=w2238:dbl)
            n991 = Select(t=w2244, s=w2246, f=w2235) -> (s? t:f=w2239:dbl)
            n992 = call "Volt to I16.vi"("Voltage In"=w2239) -> ("I16 Voltage Out"=w2242:i16)
            n993 = call "Volt to I16.vi"("Voltage In"=w2238) -> ("I16 Voltage Out"=w2241:i16)
            n994 = xnode "Read/Write Control"("FPGA VI Reference In"=w2255, "error in"=w2254, "AI to FIFO"=w2251, "APD to FIFO"=w2251, "Start scan (MCL)"=w2251, "AO1"=w2242, "AO2"=w2241) -> ("FPGA VI Reference Out"=w2253:T18, "error out"=w2252:errorcluster)
          }
        }
        "Initial Y" <- w2204
        "Initial X" <- w2203
        n995 = local write "Tab Control 6"(T3."Imaging" ("Tab Control 6")) -> ()
        "wait to reset values" <- w2205
      }
    }
    n996 = local read "Trap Pos Elements/DMA read"() -> (w1563:u32)
    n997 = local read "Trap AI Elements/DMA read"() -> (w1638:u32)
    n998 = local read "APD Elements/DMA read"() -> (w1604:u32)
    n999 = xnode "Get APD Data"("FPGA VI Reference In"=w1567, "error in"=w1566, "Number of Elements"=w1604, "Timeout (ms)"=-1) -> ("Data"=w1603:u32[], "Elements Remaining"=→"APD FIFO Elements Remaining":u32)  [unwired: 2 out]
    n1000 = xnode "Invoke Method"("FPGA VI Reference In"=w1567, "error in"=w1566, "Number of Elements"=w1563, "Timeout (ms)"=-1) -> ("Data"=w1526:u16[], "Elements Remaining"=→"Trap Pos FIFO El Remaining":u32)  [unwired: 2 out]
    n1001 = xnode "Get Trap Data"("FPGA VI Reference In"=w1567, "error in"=w1566, "Number of Elements"=w1638, "Timeout (ms)"=-1 ("Timeout")) -> ("FPGA VI Reference Out"=w1461:T18, "error out"=w1460:errorcluster, "Data"=w1527:i16[], "Elements Remaining"=w1761:u32)
    "FIFO El. Rem." <- w1761
    n1002 = local read "Trap AI FIFO Depth"() -> (w1763:u32)
    n1003 = Subtract(x=w1763, y=w1638) -> (x-y=w1762:u32)
    n1004 = Decimate 1D Array(w1526) -> (w1523:u16[], w1525:u16[], w1524:u16[])
    n1005 = Divide(x=w1761, y=w1762) -> (x/y=w1760:dbl)
    "Buffer Status" <- w1760
    n1006 = To Unsigned Long Integer(number=w1523) -> (unsigned 32bit integer=w1522:u32[])
    n1007 = Join Numbers(hi=w1525, lo=w1524) -> ((hi.lo)=w1521:u32[])
    n1008 = Equal?(x=w1760, y=1.0) -> (x = y?=w1758:bool)
    n1009 = Join Numbers(hi=w1522, lo=w1521) -> ((hi.lo)=w1515:u64[])
    n1010 = call "IR AOM word to freq - vec.vi"("Frequency Word In (double vec)"=w1515) -> ("Frequency Out"=w1562:dbl[])
    n1011 = case "Alert buffer overflow" shown="True" w1758 {
      frame False {
      }
      frame True {
        n1012 = call <vilib>:"Beep.vi"() -> ()  [unwired: 3 in, 9 out]
        "Overflow (data lost)" <- TRUE ("Overflow (data lost)")
      }
    }
    n1013 = Decimate 1D Array(w1562) -> (w1561:dbl[], w1560:dbl[])
    n1014 = Build Array(w1561, w1560) -> (w1559:dbl[][])
    n1015 = local read "Trap Sets"() -> (w1637:u32)
    n1016 = case "Deinterlace trap data, average down PSD" shown="2" w1637 {
      tunnel: w1527 -> [w2292 w2357]
      tunnel: [w2289 w2354] -> w1630
      tunnel: [w2292 w2356] -> w1518
      tunnel: "Detector Type" -> [w2291 w2352]
      tunnel: [w2290 w2355] -> w1629
      tunnel: [w2288 w2353] -> w1735
      frame 1, Default {
        n1017 = Divide(x=w2292, y=3276.7) -> (x/y=w2293:dbl[])
        n1018 = Decimate 1D Array(w2293) -> (w2302:dbl[], w2301:dbl[], w2300:dbl[], w2299:dbl[], w2298:dbl[], w2297:dbl[], w2296:dbl[], w2295:dbl[])
        n1019 = case shown="\"IR-QPD + PSD + FB-QPD position\"" w2291 {
          tunnel: w2302 -> [w2326 w2351]
          tunnel: w2301 -> [w2325 w2350]
          tunnel: w2300 -> [w2310 w2328]
          tunnel: w2299 -> [w2311 w2338]
          tunnel: w2298 -> [w2324 w2349]
          tunnel: w2297 -> [w2323 w2348]
          tunnel: w2296 -> [w2307 w2329]
          tunnel: w2295 -> [w2306 w2327]
          tunnel: [w2305 w2335] -> w2290
          tunnel: [w2304 w2334] -> w2289
          tunnel: [w2303 w2333] -> w2288
          frame "IR-QPD + PSD + FB-QPD", Default {
            w2303 = 0  # Channel pattern
            n1020 = Divide(x=w2326, y=w2311) -> (x/y=w2313:dbl[])
            n1021 = Divide(x=w2325, y=w2311) -> (x/y=w2312:dbl[])
            n1022 = Divide(x=w2324, y=w2307) -> (x/y=w2309:dbl[])
            n1023 = Divide(x=w2323, y=w2306) -> (x/y=w2308:dbl[])
            n1024 = Build Array(w2313, w2312, w2311, w2310, w2309, w2308, w2307, w2306) -> (w2304:dbl[][])
            n1025 = Bundle("T1 Y", "T1 X", "T1 Sum", "FB Sum", "PSD Y", "PSD X", "PSD Y Sum", "PSD X Sum") -> (w2322:T36)  [unwired: 1 out]
            n1026 = Cluster To Array(cluster=w2322) -> (array=w2305:string[])
          }
          frame "IR-QPD + PSD + FB-QPD position" {
            w2333 = 3  # Channel pattern
            n1027 = Negate(x=w2329) -> (-x=w2330:dbl[])
            n1028 = Divide(x=w2351, y=w2338) -> (x/y=w2340:dbl[])
            n1029 = Divide(x=w2350, y=w2338) -> (x/y=w2339:dbl[])
            n1030 = Divide(x=w2349, y=w2329) -> (x/y=w2337:dbl[])
            n1031 = Divide(x=w2348, y=w2330) -> (x/y=w2336:dbl[])
            n1032 = Build Array(w2340, w2339, w2338, w2327, w2328, w2337, w2336, w2329) -> (w2334:dbl[][])
            n1033 = Bundle("T1 Y", "T1 X", "T1 Sum", "FB X", "FB Sum", "PSD Y", "PSD X", "PSD Y Sum") -> (w2347:T36)  [unwired: 1 out]
            n1034 = Cluster To Array(cluster=w2347) -> (array=w2335:string[])
          }
        }
      }
      frame 2 {
        n1035 = case shown="\"IR-QPD + PSD + FB-QPD X position\"" w2352 {
          tunnel: w2357 -> [w2419 w2486 w2557]
          tunnel: [w2358 w2477 w2488] -> w2356
          tunnel: [w2385 w2468 w2535] -> w2355
          tunnel: [w2384 w2431 w2502] -> w2354
          tunnel: [w2378 w2466 w2533] -> w2353
          frame "IR-QPD + PSD + FB-QPD", Default {
            w2378 = 1  # Channel pattern
            # "time average x2 the 4th signal and the 4 psd signals (detection laser)"
            # "deinterlace 3 signals from qpd"
            n1036 = Decimate 1D Array(w2419) -> (w2418:i16[], w2417:i16[], w2383:i16[], w2416:i16[], w2406:i16[], w2404:i16[], w2403:i16[], w2401:i16[])
            n1037 = Decimate 1D Array(w2383) -> (w2382:i16[], w2381:i16[])
            n1038 = Decimate 1D Array(w2418) -> (w2415:i16[], w2387:i16[])
            n1039 = Decimate 1D Array(w2417) -> (w2414:i16[], w2412:i16[])
            n1040 = Decimate 1D Array(w2416) -> (w2413:i16[], w2411:i16[])
            n1041 = call "downsample 1D array - double.vi"("Ave N"=2.0, "Array In"=w2406) -> ("Array Out"=w2405:dbl[])  [unwired: 1 out]
            n1042 = call "downsample 1D array - double.vi"("Ave N"=2.0, "Array In"=w2404) -> ("Array Out"=w2386:dbl[])  [unwired: 1 out]
            n1043 = call "downsample 1D array - double.vi"("Ave N"=2.0, "Array In"=w2403) -> ("Array Out"=w2402:dbl[])  [unwired: 1 out]
            n1044 = call "downsample 1D array - double.vi"("Ave N"=2.0, "Array In"=w2401) -> ("Array Out"=w2400:dbl[])  [unwired: 1 out]
            n1045 = Interleave 1D Arrays(w2415, w2414, w2413, w2387, w2412, w2411, w2382, w2381, w2405, w2386, w2402, w2400) -> (w2399:dbl[])
            n1046 = Divide(x=w2399, y=3276.7) -> (x/y=w2398:dbl[])
            n1047 = Decimate 1D Array(w2398) -> (w2397:dbl[], w2396:dbl[], w2395:dbl[], w2394:dbl[], w2393:dbl[], w2392:dbl[], w2380:dbl[], w2379:dbl[], w2391:dbl[], w2390:dbl[], w2389:dbl[], w2388:dbl[])
            n1048 = Divide(x=w2397, y=w2395) -> (x/y=w2365:dbl[])
            n1049 = Divide(x=w2396, y=w2395) -> (x/y=w2364:dbl[])
            n1050 = Divide(x=w2394, y=w2392) -> (x/y=w2363:dbl[])
            n1051 = Divide(x=w2393, y=w2392) -> (x/y=w2362:dbl[])
            n1052 = Divide(x=w2391, y=w2389) -> (x/y=w2361:dbl[])
            n1053 = Divide(x=w2390, y=w2388) -> (x/y=w2360:dbl[])
            n1054 = Build Array(w2365, w2364, w2395, w2363, w2362, w2392, w2380, w2379, w2361, w2360, w2389, w2388) -> (w2384:dbl[][])
            n1055 = Bundle("T1 Y", "T1 X", "T1 Sum", "T2 Y", "T2 X", "T2 Sum", "T1 FB Sum", "T2 FB Sum", "PSD Y", "PSD X", "PSD Y Sum", "PSD X Sum") -> (w2366:T37)  [unwired: 1 out]
            n1056 = To Word Integer(number=w2399) -> (16bit integer=w2358:i16[])
            n1057 = Cluster To Array(cluster=w2366) -> (array=w2385:string[])
          }
          frame "IR-QPD + PSD + FB-QPD X position" {
            w2466 = 2  # Channel pattern
            # "time average x2 the 3 psd signals (detection laser)"
            # "deinterlace 3 signals from qpds"
            n1058 = Decimate 1D Array(w2486) -> (w2485:i16[], w2484:i16[], w2467:i16[], w2483:i16[], w2429:i16[], w2426:i16[], w2423:i16[], w2454:i16[])
            n1059 = Decimate 1D Array(w2467) -> (w2452:i16[], w2450:i16[])
            n1060 = Decimate 1D Array(w2485) -> (w2482:i16[], w2469:i16[])
            n1061 = Decimate 1D Array(w2484) -> (w2481:i16[], w2479:i16[])
            n1062 = Decimate 1D Array(w2483) -> (w2480:i16[], w2478:i16[])
            n1063 = Decimate 1D Array(w2454) -> (w2453:i16[], w2451:i16[])
            n1064 = call "downsample 1D array - I16.vi"("Ave N"=2.0, "Array In"=w2429) -> ("Array Out"=w2427:i16[])  [unwired: 1 in]
            n1065 = call "downsample 1D array - I16.vi"("Ave N"=2.0, "Array In"=w2423) -> ("Array Out"=w2421:i16[])  [unwired: 1 in]
            n1066 = call "downsample 1D array - I16.vi"("Ave N"=2.0, "Array In"=w2426) -> ("Array Out"=w2424:i16[])  [unwired: 1 in]
            n1067 = Interleave 1D Arrays(w2482, w2481, w2480, w2469, w2479, w2478, w2453, w2452, w2451, w2450, w2427, w2424, w2421) -> (w2477:i16[])
            n1068 = Divide(x=w2477, y=3276.7) -> (x/y=w2476:dbl[])
            n1069 = Decimate 1D Array(w2476) -> (w2475:dbl[], w2474:dbl[], w2473:dbl[], w2472:dbl[], w2471:dbl[], w2470:dbl[], w2442:dbl[], w2440:dbl[], w2439:dbl[], w2437:dbl[], w2436:dbl[], w2435:dbl[], w2432:dbl[])
            n1070 = Negate(x=w2432) -> (-x=w2430:dbl[])
            n1071 = Divide(x=w2436, y=w2432) -> (x/y=w2434:dbl[])
            n1072 = Divide(x=w2435, y=w2430) -> (x/y=w2433:dbl[])
            n1073 = Divide(x=w2475, y=w2473) -> (x/y=w2458:dbl[])
            n1074 = Divide(x=w2474, y=w2473) -> (x/y=w2457:dbl[])
            n1075 = Divide(x=w2472, y=w2470) -> (x/y=w2456:dbl[])
            n1076 = Divide(x=w2471, y=w2470) -> (x/y=w2455:dbl[])
            n1077 = Divide(x=w2442, y=w2440) -> (x/y=w2441:dbl[])
            n1078 = Divide(x=w2439, y=w2437) -> (x/y=w2438:dbl[])
            n1079 = Build Array(w2458, w2457, w2473, w2456, w2455, w2470, w2441, w2440, w2438, w2437, w2434, w2433, w2432) -> (w2431:dbl[][])
            n1080 = Bundle("T1 Y", "T1 X", "T1 Sum", "T2 Y", "T2 X", "T2 Sum", "T1 FB X", "T1 FB Sum", "T2 FB X", "T2 FB Sum", "PSD Y", "PSD X", "PSD Y Sum") -> (w2459:T38)  [unwired: 1 out]
            n1081 = Cluster To Array(cluster=w2459) -> (array=w2468:string[])
          }
          frame "IR-QPD + PSD + FB-QPD XY positions" {
            w2533 = 4  # Channel pattern
            # "time average x2 the 3 psd signals (detection laser)"
            # "deinterlace 3 signals from qpds"
            n1082 = Decimate 1D Array(w2557) -> (w2556:i16[], w2555:i16[], w2534:i16[], w2554:i16[], w2500:i16[], w2546:i16[], w2545:i16[], w2522:i16[])
            n1083 = Decimate 1D Array "Feedback Sum"(w2534) -> (w2518:i16[], w2516:i16[])
            n1084 = Decimate 1D Array "QPD Y"(w2556) -> (w2553:i16[], w2536:i16[])
            n1085 = Decimate 1D Array "QPD X"(w2555) -> (w2552:i16[], w2550:i16[])
            n1086 = Decimate 1D Array "Feedback Y"(w2500) -> (w2499:i16[], w2498:i16[])
            n1087 = Decimate 1D Array "QPD Sum"(w2554) -> (w2551:i16[], w2549:i16[])
            n1088 = Decimate 1D Array "Feedback X"(w2522) -> (w2519:i16[], w2517:i16[])
            n1089 = call "downsample 1D array - double.vi"("Ave N"=2.0, "Array In"=w2546) -> ("Array Out"=w2521:dbl[])  [unwired: 1 out]
            n1090 = call "downsample 1D array - double.vi"("Ave N"=2.0, "Array In"=w2545) -> ("Array Out"=w2520:dbl[])  [unwired: 1 out]
            n1091 = Interleave 1D Arrays(w2553, w2552, w2551, w2536, w2550, w2549, w2499, w2519, w2518, w2498, w2517, w2516, w2521, w2520) -> (w2544:dbl[])
            n1092 = Divide(x=w2544, y=3276.7) -> (x/y=w2543:dbl[])
            n1093 = Decimate 1D Array(w2543) -> (w2542:dbl[], w2541:dbl[], w2540:dbl[], w2539:dbl[], w2538:dbl[], w2537:dbl[], w2495:dbl[], w2509:dbl[], w2493:dbl[], w2494:dbl[], w2507:dbl[], w2491:dbl[], w2505:dbl[], w2503:dbl[])
            n1094 = Negate(x=w2503) -> (-x=w2501:dbl[])
            n1095 = Divide(x=w2505, y=w2501) -> (x/y=w2504:dbl[])
            n1096 = Divide(x=w2494, y=w2491) -> (x/y=w2490:dbl[])
